vi "Single Tone Measurements - Custom.vi"() -> ()   [LabVIEW 2020]
doc: "Demonstrates the measurement of the frequency and amplitude of the input signal. This example gives you the ability to narrow the search to a particular frequency using the advanced search criteria."
uses:
  <vilib>/measure/matone.llb/Extract Single Tone Information.vi
  <vilib>/measure/NI_MAPro.lvlib
panel:
  out "Amplitude error (ppm)":dbl(knob) scale=0.0..10.0
  out "Frequency error (ppm)":dbl(knob) scale=0.0..10.0
  in  "Noise \"bitVolt\"":dbl(slide)=-14.89795918367347
  in  "export mode":u16(ring)=1 items=["none", "input signal", "detected signal", "residual signal"]
  in  "advanced search":T1={"approx freq. (optional)"=-1.0, "search (+/- % of Fsampl.)"=1.0}
  in  "Block size":i32=200
  out "Amplitude Result":dbl format="%_6g"
  out "Frequency Result":dbl
  out "Exported signal spectrum (dBV)":T2(graph)
  in  "second tone":bool
  in  "Stop":bool
  out "Exported time signal":waveform(dbl)(graph)
  in  "Amplitude (V)":dbl=1.0
  in  "Frequency (Hz)":dbl=8067.89
  in  "Fs (Hz)":dbl=51200.0
  # "Input Signal"
  # "Analysis Results"
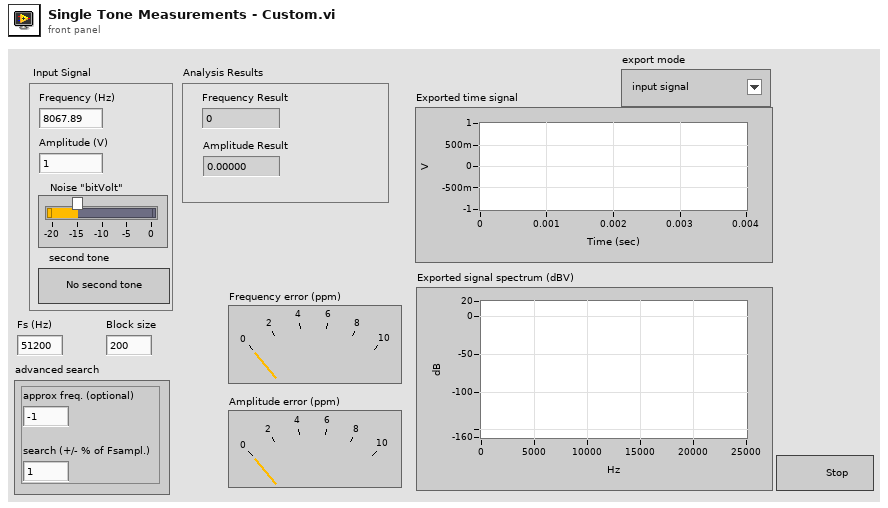
[diagram p1: front panel]
types:
  T1 = cluster{"approx freq. (optional)":dbl, "search (+/- % of Fsampl.)":dbl}
  T2 = cluster{"f0":dbl, "df":dbl, "dB Spectrum (Hann)":dbl[]}
  T3 = cluster{"exported time signal":waveform(dbl), "exported spectrum (dB)":cluster{"f0":dbl, "df":dbl, "dB Spectrum (Hann)":dbl[]}}
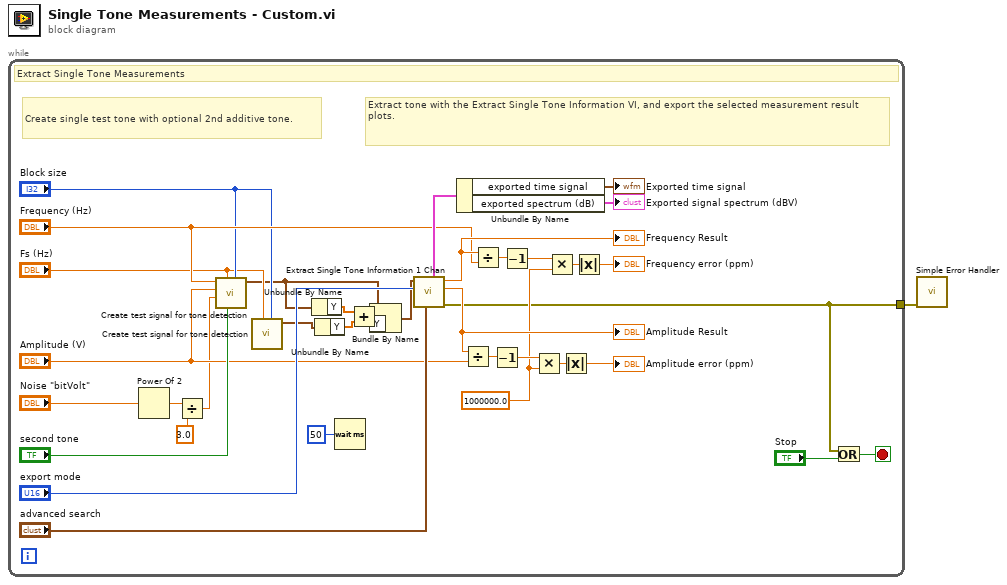
[diagram p0: block diagram]
diagram:
  n1 = while {
    tunnel: [w11] -> w1
    stop <- w12 stop-if-true
    w13 = 1000000.0
    # "Extract tone with the Extract Single Tone Information VI, and export the selected measurement result plots."
    # "Create single test tone with optional 2nd additive tone."
    # "Extract Single Tone Measurements"
    n2 = Power Of 2(x="Noise \"bitVolt\"") -> (2^x=w35:dbl)
    n3 = Divide(x=w35, y=3.0) -> (x/y=w15:dbl)
    n4 = call "Create test signal for tone detection.vi"("block size"="Block size", "second tone"="second tone", "sampling frequency (Hz)"="Fs (Hz)", "Noise level (Vrms)"=w15, "Tone amplitude"="Amplitude (V)", "Tone frequency (Hz)"="Frequency (Hz)") -> ("Test signal"=w3:waveform(dbl))  [unwired: 5 in]
    n5 = call "Create test signal for tone detection.vi"("block size"="Block size", "sampling frequency (Hz)"="Fs (Hz)") -> ("Test signal"=w7:waveform(dbl))  [unwired: 9 in]
    n6 = Unbundle By Name(w3) -> ("Y"=w6:dbl[])
    n7 = Unbundle By Name(w7) -> ("Y"=w5:dbl[])
    n8 = Wait (ms)(milliseconds to wait=u32 50) -> ()  [unwired: 1 out]
    n9 = Add(x=w6, y=w5) -> (x+y=w4:dbl[])
    n10 = Bundle By Name(cluster=w3, "Y"=w4) -> (w2:waveform(dbl))
    n11 = call-poly <vilib>:"Extract Single Tone Information 1 Chan.vi"("advanced search"="advanced search", "export mode"="export mode", "time signal in"=w2) -> ("error out"=w11:errorcluster, "detected amplitude"=w26:dbl, "detected frequency"=w27:dbl, "exported signals"=w23:T3)  [unwired: 3 in, 2 out]
    "Frequency Result" <- w27
    "Amplitude Result" <- w26
    n12 = Unbundle By Name(w23) -> ("exported time signal"=→"Exported time signal":waveform(dbl), "exported spectrum (dB)"=→"Exported signal spectrum (dBV)":T2)
    n13 = Divide(x=w26, y="Amplitude (V)") -> (x/y=w29:dbl)
    n14 = Divide(x=w27, y="Frequency (Hz)") -> (x/y=w34:dbl)
    n15 = Decrement(x=w29) -> (x-1=w30:dbl)
    n16 = Decrement(x=w34) -> (x-1=w33:dbl)
    n17 = Multiply(x=w30, y=w13) -> (x*y=w31:dbl)
    n18 = Multiply(x=w33, y=w13) -> (x*y=w32:dbl)
    n19 = Absolute Value(x=w31) -> (abs(x)=→"Amplitude error (ppm)":dbl)
    n20 = Absolute Value(x=w32) -> (abs(x)=→"Frequency error (ppm)":dbl)
    n21 = Or(x=w11, y="Stop") -> (x .or. y?=w12:bool)
  }
  n22 = call <vilib>:"Simple Error Handler.vi"("error in (no error)"=w1) -> ()  [unwired: 4 in, 5 out]
